vi "Trapezoidal Test.vi"(9 "Function Parameters":cluster{"Prefactor":dbl, "Power":dbl}={"Prefactor"=5.0, "Power"=4.0}, 10 "Digitizing Parameters":T1={"Number of Samples"=0, "Lower Limit"=0.0, "Upper Limit"=1.0}) -> (2 "Value of Integral":dbl format="%.10g")   [LabVIEW 2017]
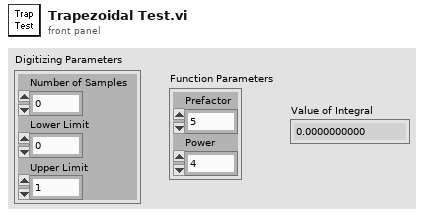
[diagram p1: front panel]
types:
  T1 = cluster{"Number of Samples":i32, "Lower Limit":dbl, "Upper Limit":dbl}
  T2 = cluster{"X Array":dbl[], "Y Array":dbl[], "delta_x":dbl}
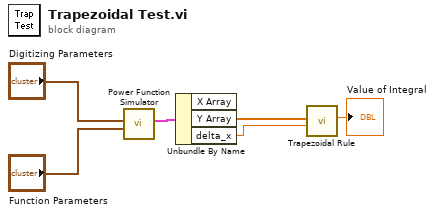
[diagram p0: block diagram]
diagram:
  n1 = call "Power Function Simulator.vi"("Function Parameters"="Function Parameters", "Digitizing Parameters"="Digitizing Parameters") -> ("Output Cluster"=w4:T2)  [unwired: 9 in]
  n2 = Unbundle By Name(w4) -> ("Y Array"=w3:dbl[], "delta_x"=w2:dbl)  [unwired: 1 out]
  n3 = call "Trapezoidal Rule.vi"("Delta_x"=w2, "y array"=w3) -> ("Value of Integral"=→"Value of Integral":dbl)  [unwired: 9 in]
